vi "模块启用配置框.vi"() -> ()   [LabVIEW 2022 SP3]
uses:
  <vilib>/Utility/config.llb/NI_LVConfig.lvlib
  <userlib>/_OpenG.lib/variantconfig/variantconfig.llb/openg_variant_configuration_file.lvlib
panel:
  in  "旁路系统启用":bool caption="启用"
  in  "综合生物毒性启用":bool caption="启用"
  in  "雷达流速仪启用":bool caption="启用"
  in  "ADCP启用":bool caption="启用"
  in  "挥发酚启用":bool caption="启用"
  in  "重金属启用":bool caption="启用"
  in  "运维打卡启用":bool caption="启用"
  in  "氟化物连接配置":T1={"启用"=FALSE, "连接类型"=enum."串口", "串口"="", "波特率"=115200, "IP"="", "PORT"="502"} {"波特率" items=["115200"=115200, "9600"=9600]}
  in  "加标回收模块版本":T2=enum."V4"
  in  "多参数模块版本":T3=enum."集成式多参"
  in  "总氮模块版本":T4=enum."V3"
  in  "总磷模块版本":T4=enum."V3"
  in  "加标回收连接配置":T1={"启用"=FALSE, "连接类型"=enum."串口", "串口"="", "波特率"=115200, "IP"="", "PORT"="502"} {"波特率" items=["115200"=115200, "9600"=9600]}
  in  "多参数连接配置":T1={"启用"=FALSE, "连接类型"=enum."串口", "串口"="", "波特率"=115200, "IP"="", "PORT"="502"} {"波特率" items=["115200"=115200, "9600"=9600]}
  in  "CODcr连接配置":T1={"启用"=FALSE, "连接类型"=enum."串口", "串口"="", "波特率"=115200, "IP"="", "PORT"="502"} {"波特率" items=["115200"=115200, "9600"=9600]}
  in  "CODMn连接配置":T1={"启用"=FALSE, "连接类型"=enum."串口", "串口"="", "波特率"=115200, "IP"="", "PORT"="502"} {"波特率" items=["115200"=115200, "9600"=9600]}
  in  "总氮连接配置":T1={"启用"=FALSE, "连接类型"=enum."串口", "串口"="", "波特率"=115200, "IP"="", "PORT"="502"} {"波特率" items=["115200"=115200, "9600"=9600]}
  in  "总磷连接配置":T1={"启用"=FALSE, "连接类型"=enum."串口", "串口"="", "波特率"=115200, "IP"="", "PORT"="502"} {"波特率" items=["115200"=115200, "9600"=9600]}
  in  "氨氮连接配置":T1={"启用"=FALSE, "连接类型"=enum."串口", "串口"="", "波特率"=115200, "IP"="", "PORT"="502"} {"波特率" items=["115200"=115200, "9600"=9600]}
  in  "进样类型":T5={"氨氮采样杯采样"=TRUE, "总磷采样杯采样"=TRUE, "总氮采样杯采样"=TRUE, "CODMn采样杯采样"=TRUE, "CODcr采样杯采样"=TRUE, "氟化物采样杯采样"=TRUE, "挥发酚采样杯采样"=TRUE}
  in  "CODcr模块版本":T6
  in  "加载配置":bool
  in  "河水净化启用":bool caption="启用"
  in  "流量计启用":bool caption="启用"
  in  "超标留样启用":bool caption="启用"
  in  "氨氮模块版本":T4=enum."V3"
  in  "设备类型":T7=enum."浮船"
  in  "采配水模块类型":T8=enum."V4"
  in  "CODMn模块版本":T9
  in  "数据库类型":T10
  in  "模块配置类型":T11
  in  "取消":bool
  in  "确认":bool
  # "模块启用配置"
  # "说明:\n选择所需要启动的模块,并按确认,软件将重启生效."
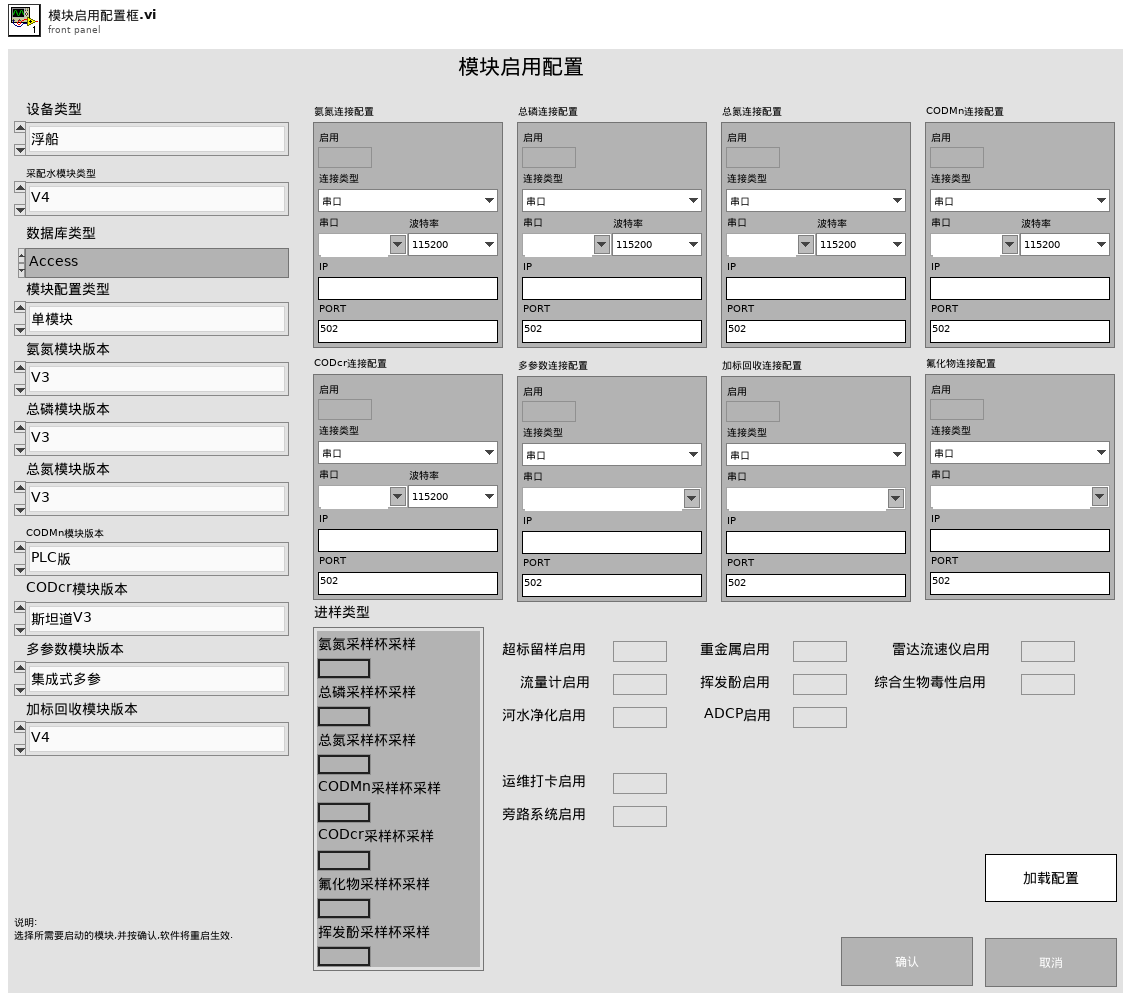
[diagram p1: front panel]
types:
  T1 = typedef "连接配置.ctl" = cluster{"启用":bool, "连接类型":enum16{"串口", "TCP"}, "串口":string, "波特率":u32, "IP":string, "PORT":string}
  T2 = typedef "加标回收模块版本.ctl" = enum16{"V1", "V2", "V4"}
  T3 = typedef "多参数模块版本.ctl" = enum16{"原位多参数", "集成式多参"}
  T4 = typedef "氨氮总磷总氮模块版本.ctl" = enum16{"V2", "V3"}
  T5 = cluster{"氨氮采样杯采样":bool, "总磷采样杯采样":bool, "总氮采样杯采样":bool, "CODMn采样杯采样":bool, "CODcr采样杯采样":bool, "氟化物采样杯采样":bool, "挥发酚采样杯采样":bool}
  T6 = typedef "CODcr模块版本.ctl" = enum16{"斯坦道V3", "点创"}
  T7 = typedef "设备类型.ctl" = enum16{"微站", "固定站", "浮船"}
  T8 = typedef "采配水类型.ctl" = enum16{"V1", "V2", "V3", "V4", "室内V1", "室内V2", "固定站V1", "固定站V2", "浮船V1", "浮船V2", "养殖尾水", "广东华南所"}
  T9 = typedef "CODMn模块版本.ctl" = enum16{"PLC版", "单片机版", "通用流路版本"}
  T10 = typedef "数据库类型.ctl" = enum16{"Access", "SQLite"}
  T11 = typedef "模块配置类型.ctl" = enum16{"单模块", "总磷总氮二合一模块", "氨氮总磷二合一模块"}
  T12 = cluster{"氨氮采样杯采样":bool, "总磷采样杯采样":bool, "总氮采样杯采样":bool, "CODMn采样杯采样":bool, "CODcr采样杯采样":bool, "氟化物采样杯采样":bool, "氟化物采样杯采样 2":bool}
  T13 = cluster{"总磷总氮启用":bool, "MB通信方式选择":enum16{"串口", "TCP"}, "VISA Resource":refnum<visa-resource-name>, "波特率":u32, "IP":string, "PORT":string}
  T14 = cluster{"质控单元启用":bool, u16, "COM Port":refnum<visa-resource-name>, "Baud Rate (bps)":u32, "IP Address":string, string}
  T15 = cluster{"氟化物启用":bool, "MB通信方式选择":enum16{"串口", "TCP"}, "VISA Resource":refnum<visa-resource-name>, "波特率":u32, "IP":string, "PORT":string}
  T16 = cluster{"总氮启用":bool, "MB通信方式选择":enum16{"串口", "TCP"}, "VISA Resource":refnum<visa-resource-name>, "波特率":u32, "IP":string, "PORT":string}
  T17 = cluster{"多参数启用":bool, "MB通信方式选择":enum16{"串口", "TCP"}, "VISA Resource":refnum<visa-resource-name>, "波特率":u32, "IP":string, "PORT":string}
  T18 = cluster{"多参数启用":bool, "连接方式":u16, "VISA资源名称":refnum<visa-resource-name>, "波特率":u32, "IP":string, string}
  T19 = cluster{"氨氮启用":bool, "MB通信方式选择":enum16{"串口", "TCP"}, "VISA Resource":refnum<visa-resource-name>, "波特率":u32, "IP":string, "PORT":string}
  T20 = cluster{"CODcr启用":bool, "MB通信方式选择":enum16{"串口", "TCP"}, "VISA Resource":refnum<visa-resource-name>, "波特率":u32, "IP":string, "PORT":string}
  T21 = cluster{"baud rate (bps)":u32, "stop bits":u16, "parity":u16, "flow control":u16, "timeout":u32, "retries":i32}
  T22 = cluster{"CODMn启用":bool, "MB通信方式选择":enum16{"串口", "TCP"}, "VISA resource name":refnum<visa-resource-name>, "baud rate (bps)":u32, "IP":string, "PORT":string}
  T23 = cluster{"CODMn启用":bool, "MB通信方式选择":enum16{"串口", "TCP"}, "VISA Resource":refnum<visa-resource-name>, "波特率":u32, "IP":string, "PORT":string}
  T24 = typedef "配置表选择.ctl" = enum16{"微站常规九参总磷总氮二合一", "微站常规八参氨氮总磷二合一", "微站常规九参", "微站常规八参", "固定站常规九参（TCP连接）", "固定站常规九参（串口连接）", "浮船常规九参总磷总氮二合一", "浮船常规九参"}
  T25 = typedef "模块配置表.ctl" = cluster{"设备类型":T7, "采配水模块类型":T8, "数据库类型":T10, "模块配置类型":T11, "氨氮模块版本":T4, "总磷模块版本":T4, "总氮模块版本":T4, "CODMn模块版本":T9, "CODcr模块版本":T6, "多参数模块版本":T3, "加标回收模块版本":T2, "氨氮连接配置":T1, "总磷连接配置":T1, "总氮连接配置":T1, "CODMn连接配置":T1, "CODcr连接配置":T1, "多参数连接配置":T1, "加标回收连接配置":T1, "超标留样启用":bool, "流量计启用":bool, "河水净化启用":bool, "进样类型":cluster{"氨氮采样杯采样":bool, "总磷采样杯采样":bool, "总氮采样杯采样":bool, "CODMn采样杯采样":bool, "CODcr采样杯采样":bool, "氟化物采样杯采样":bool, "挥发酚采样杯采样":bool}, "氟化物连接配置":T1}
  T26 = typedef "NI_LVConfig.lvlib/Config Data RefNum.ctl" = refnum<k1>
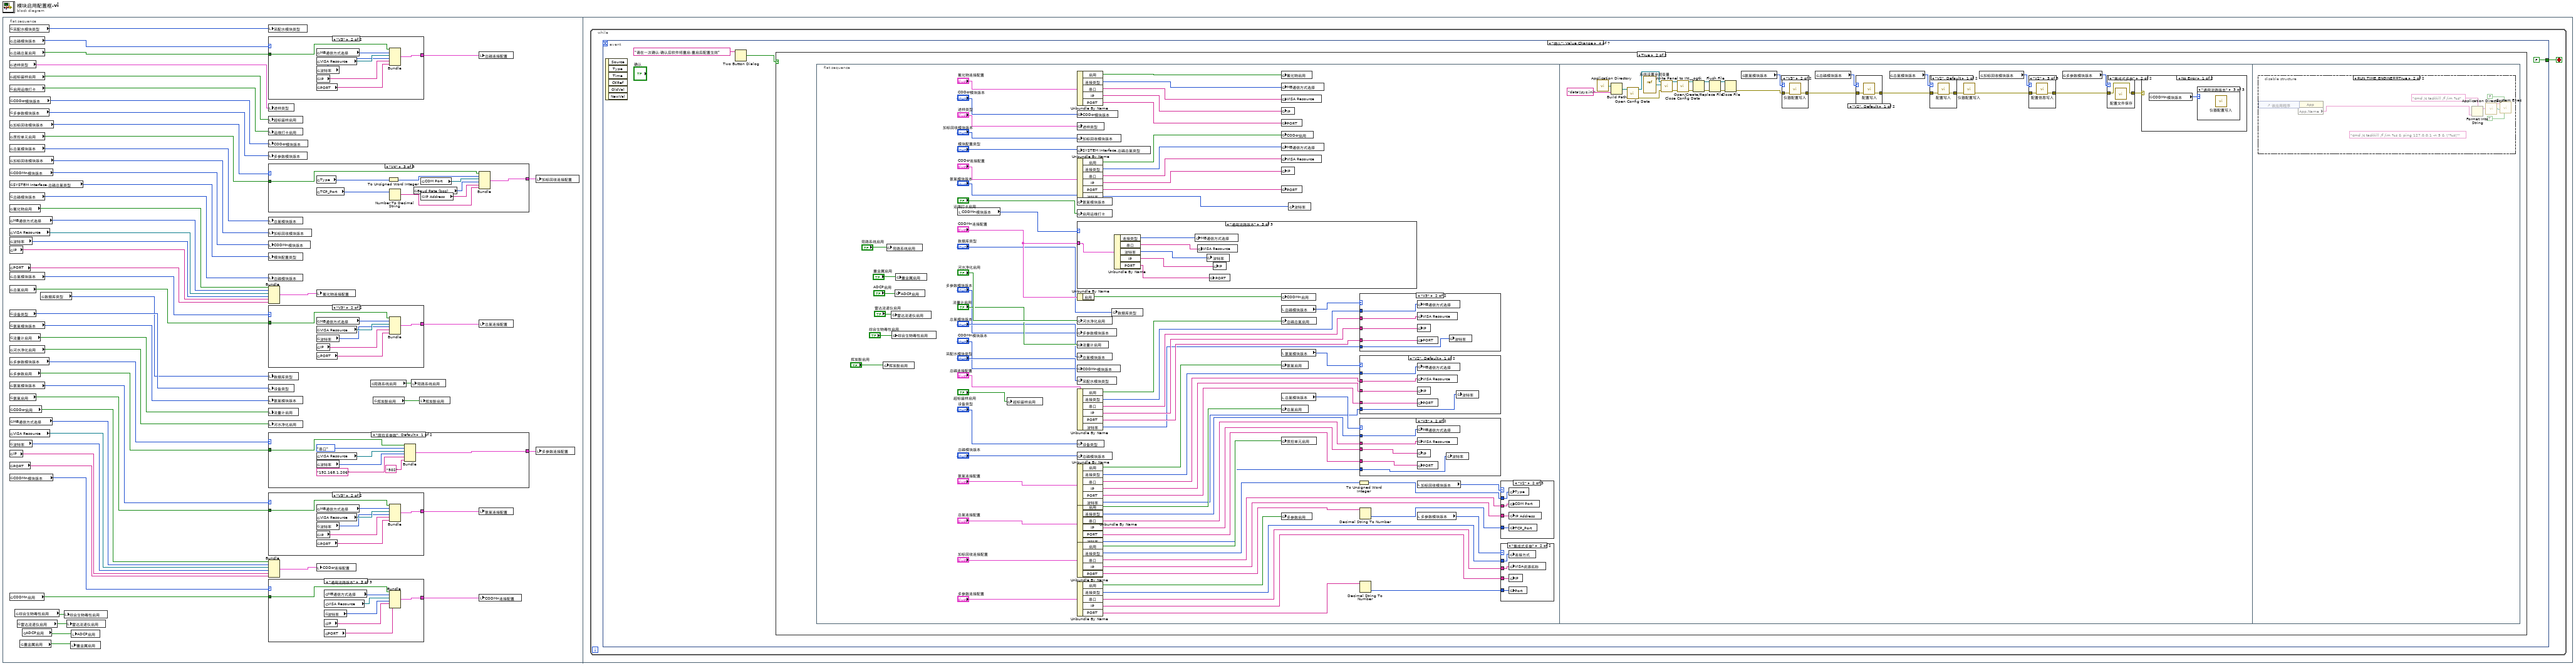
[diagram p0: block diagram]
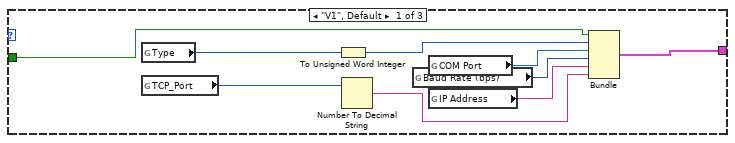
[diagram p2: hidden frame]
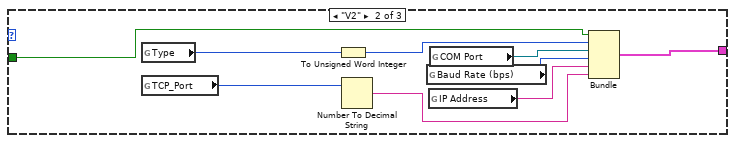
[diagram p3: hidden frame]
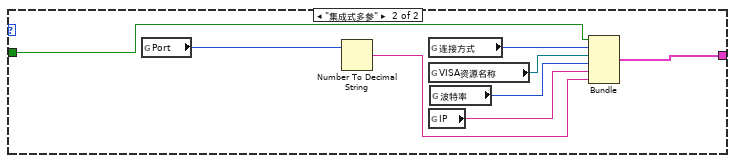
[diagram p4: hidden frame]
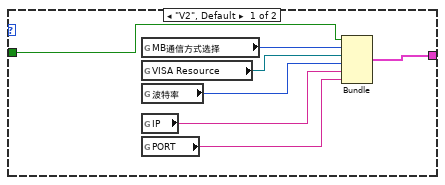
[diagram p5: hidden frame]
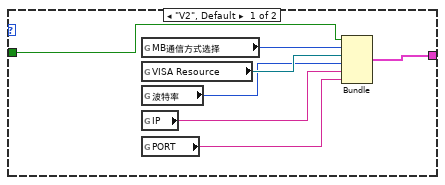
[diagram p6: hidden frame]
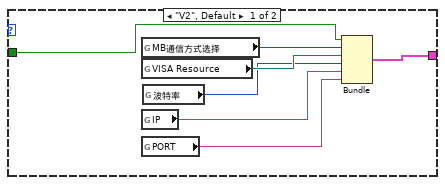
[diagram p7: hidden frame]
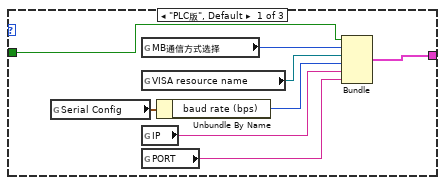
[diagram p8: hidden frame]
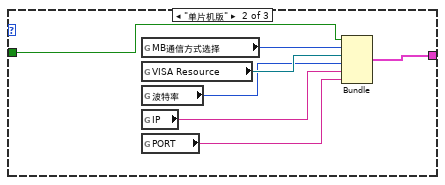
[diagram p9: hidden frame]
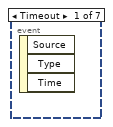
[diagram p10: hidden frame]
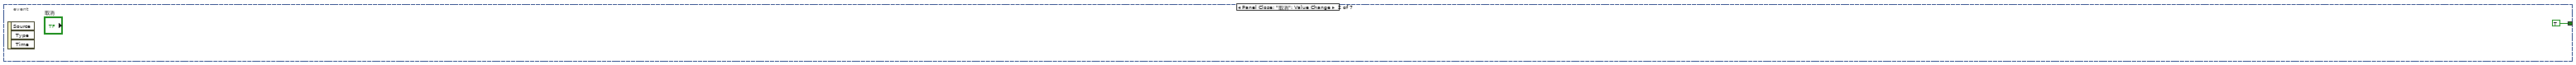
[diagram p11: hidden frame]
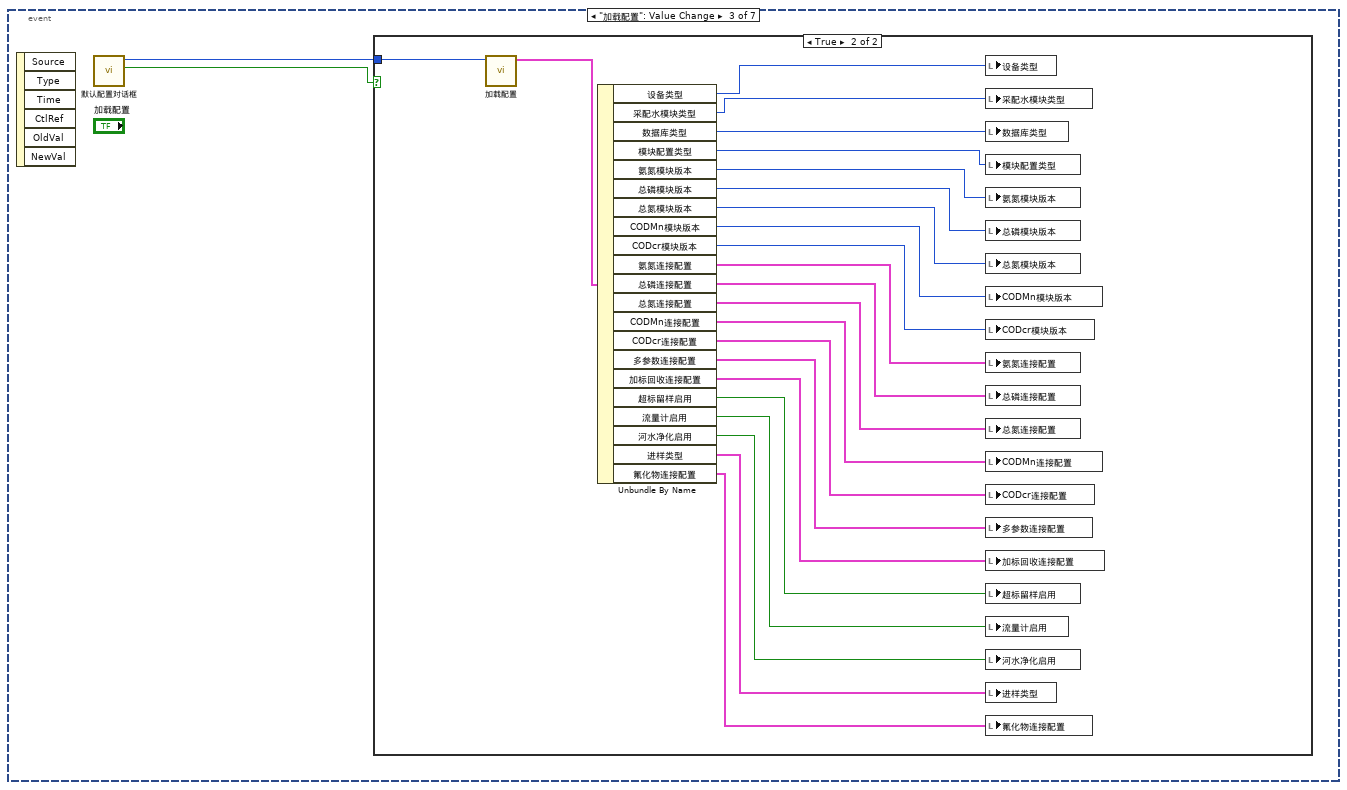
[diagram p12: hidden frame]
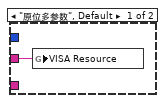
[diagram p15: hidden frame]
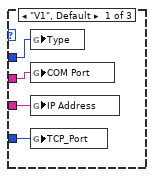
[diagram p16: hidden frame]
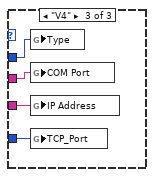
[diagram p17: hidden frame]
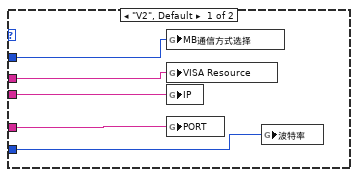
[diagram p18: hidden frame]
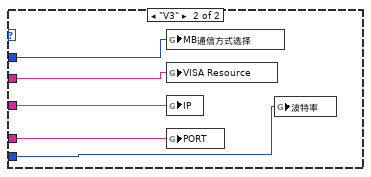
[diagram p19: hidden frame]
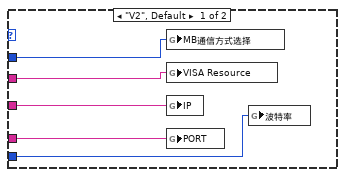
[diagram p20: hidden frame]
diagram:
  n1 = flat-sequence {
    frame #0 {
      n2 = global read "系统设置全局变量.vi" "采配水模块类型"() -> (w53:T8)
      n3 = global read "系统设置全局变量.vi" "总磷模块版本"() -> (w27:T4)
      n4 = global read "系统设置全局变量.vi" "总磷总氮启用"() -> (w25:bool)
      n5 = global read "系统设置全局变量.vi" "进样类型"() -> (w48:T5)
      n6 = global read "系统设置全局变量.vi" "超标留样启用"() -> (w47:bool)
      n7 = global read "系统设置全局变量.vi" "启用运维打卡"() -> (w11:bool)
      n8 = global read "系统设置全局变量.vi" "CODcr模块版本"() -> (w49:T6)
      n9 = global read "系统设置全局变量.vi" "多参数模块版本"() -> (w23:T3)
      n10 = global read "系统设置全局变量.vi" "加标回收模块版本"() -> (w19:T2)
      n11 = global read "系统设置全局变量.vi" "质控单元启用"() -> (w18:bool)
      n12 = global read "系统设置全局变量.vi" "总氮模块版本"() -> (w30:T4)
      n13 = global read "系统设置全局变量.vi" "加标回收模块版本"() -> (w20:T2)
      n14 = global read "系统设置全局变量.vi" "CODMn模块版本"() -> (w50:T9)
      n15 = global read "系统设置全局变量.vi" "SYSTEM Interface.总磷总氮类型"() -> (w52:T11)
      n16 = global read "系统设置全局变量.vi" "总磷模块版本"() -> (w31:T4)
      n17 = global read "系统设置全局变量.vi" "氟化物启用"() -> (w13:bool)
      n18 = global read "总磷总氮断电保存全局变量.vi" "MB通信方式选择"() -> (w14:enum16{"串口", "TCP"})
      n19 = global read "总磷总氮断电保存全局变量.vi" "VISA Resource"() -> (w15:refnum<visa-resource-name>)
      n20 = global read "总磷总氮断电保存全局变量.vi" "波特率"() -> (w4:u32)
      n21 = global read "总磷总氮断电保存全局变量.vi" "IP"() -> (w16:string)
      n22 = global read "总磷总氮断电保存全局变量.vi" "PORT"() -> (w17:string)
      n23 = global read "系统设置全局变量.vi" "总氮模块版本"() -> (w26:T4)
      n24 = global read "系统设置全局变量.vi" "总氮启用"() -> (w24:bool)
      n25 = global read "系统设置全局变量.vi" "设备类型"() -> (w54:T7)
      n26 = global read "系统设置全局变量.vi" "氨氮模块版本"() -> (w51:T4)
      n27 = global read "系统设置全局变量.vi" "流量计启用"() -> (w46:bool)
      n28 = global read "系统设置全局变量.vi" "河水净化启用"() -> (w45:bool)
      n29 = global read "系统设置全局变量.vi" "多参数模块版本"() -> (w22:T3)
      n30 = global read "系统设置全局变量.vi" "多参数启用"() -> (w21:bool)
      n31 = global read "系统设置全局变量.vi" "氨氮模块版本"() -> (w29:T4)
      n32 = global read "系统设置全局变量.vi" "氨氮启用"() -> (w28:bool)
      n33 = global read "系统设置全局变量.vi" "CODcr启用"() -> (w38:bool)
      n34 = global read "总磷总氮断电保存全局变量.vi" "MB通信方式选择"() -> (w37:enum16{"串口", "TCP"})
      n35 = global read "总磷总氮断电保存全局变量.vi" "VISA Resource"() -> (w6:refnum<visa-resource-name>)
      n36 = global read "总磷总氮断电保存全局变量.vi" "波特率"() -> (w5:u32)
      n37 = global read "总磷总氮断电保存全局变量.vi" "IP"() -> (w36:string)
      n38 = global read "总磷总氮断电保存全局变量.vi" "PORT"() -> (w35:string)
      n39 = global read "系统设置全局变量.vi" "CODMn模块版本"() -> (w41:T9)
      n40 = global read "系统设置全局变量.vi" "CODMn启用"() -> (w40:bool)
      n41 = global read "系统设置全局变量.vi" "综合生物毒性启用"() -> (w3:bool)
      n42 = global read "系统设置全局变量.vi" "雷达流速仪启用"() -> (w1:bool)
      n43 = global read "系统设置全局变量.vi" "重金属启用"() -> (w10:bool)
      n44 = global read "系统设置全局变量.vi" "ADCP启用"() -> (w7:bool)
      n45 = global read "非断电保持全局变量.vi" "数据库类型"() -> (w8:T10)
      n46 = local write "综合生物毒性启用"(w3) -> ()
      n47 = local write "雷达流速仪启用"(w1) -> ()
      n48 = local write "重金属启用"(w10) -> ()
      n49 = local write "ADCP启用"(w7) -> ()
      n50 = local write "采配水模块类型"(w53) -> ()
      n51 = case shown="\"V3\"" w27 {
        tunnel: [w112 w120] -> w43
        tunnel: w25 -> [w117 w119]
        frame "V2", Default {
          n52 = global read "总磷总氮断电保存全局变量.vi" "MB通信方式选择"() -> (w116:enum16{"串口", "TCP"})
          n53 = global read "总磷总氮断电保存全局变量.vi" "VISA Resource"() -> (w115:refnum<visa-resource-name>)
          n54 = global read "总磷总氮断电保存全局变量.vi" "波特率"() -> (w111:u32)
          n55 = global read "总磷总氮断电保存全局变量.vi" "IP"() -> (w114:string)
          n56 = global read "总磷总氮断电保存全局变量.vi" "PORT"() -> (w113:string)
          n57 = Bundle("总磷总氮启用"=w117, "MB通信方式选择"=w116, "VISA Resource"=w115, "波特率"=w111, "IP"=w114, "PORT"=w113) -> (w112:T13)  [unwired: 1 in]
        }
        frame "V3" {
          n58 = global read "总磷总氮断电保存全局变量.vi" "MB通信方式选择"() -> (w124:enum16{"串口", "TCP"})
          n59 = global read "总磷总氮断电保存全局变量.vi" "VISA Resource"() -> (w123:refnum<visa-resource-name>)
          n60 = global read "总磷总氮断电保存全局变量.vi" "波特率"() -> (w118:u32)
          n61 = global read "总磷总氮断电保存全局变量.vi" "IP"() -> (w122:string)
          n62 = global read "总磷总氮断电保存全局变量.vi" "PORT"() -> (w121:string)
          n63 = Bundle("总磷总氮启用"=w119, "MB通信方式选择"=w124, "VISA Resource"=w123, "波特率"=w118, "IP"=w122, "PORT"=w121) -> (w120:T13)  [unwired: 1 in]
        }
      }
      n64 = local write "进样类型"(w48) -> ()
      n65 = local write "超标留样启用"(w47) -> ()
      n66 = local write "运维打卡启用"(w11) -> ()
      n67 = local write "CODcr模块版本"(w49) -> ()
      n68 = local write "多参数模块版本"(w23) -> ()
      n69 = case shown="\"V4\"" w19 {
        tunnel: [w62 w71 w77] -> w32
        tunnel: w18 -> [w63 w72 w74]
        frame "V1", Default {
          n70 = global read "ZK断电保存全局变量.vi" "Type"() -> (w61:enum16{"Serial", "TCP"})
          n71 = global read "ZK断电保存全局变量.vi" "TCP_Port"() -> (w57:u16)
          n72 = To Unsigned Word Integer(number=w61) -> (unsigned 16bit integer=w60:u16)
          n73 = Number To Decimal String(number=w57) -> (decimal integer string=w56:string)  [unwired: 1 in]
          n74 = global read "ZK断电保存全局变量.vi" "Baud Rate (bps)"() -> (w55:u32)
          n75 = global read "ZK断电保存全局变量.vi" "COM Port"() -> (w59:refnum<visa-resource-name>)
          n76 = global read "ZK断电保存全局变量.vi" "IP Address"() -> (w58:string)
          n77 = Bundle("质控单元启用"=w63, w60, "COM Port"=w59, "Baud Rate (bps)"=w55, "IP Address"=w58, w56) -> (w62:T14)  [unwired: 1 in]
        }
        frame "V2" {
          n78 = global read "ZK断电保存全局变量.vi" "Type"() -> (w68:enum16{"Serial", "TCP"})
          n79 = global read "ZK断电保存全局变量.vi" "TCP_Port"() -> (w65:u16)
          n80 = To Unsigned Word Integer(number=w68) -> (unsigned 16bit integer=w70:u16)
          n81 = Number To Decimal String(number=w65) -> (decimal integer string=w69:string)  [unwired: 1 in]
          n82 = global read "ZK断电保存全局变量.vi" "Baud Rate (bps)"() -> (w64:u32)
          n83 = global read "ZK断电保存全局变量.vi" "IP Address"() -> (w66:string)
          n84 = global read "ZK断电保存全局变量.vi" "COM Port"() -> (w67:refnum<visa-resource-name>)
          n85 = Bundle("质控单元启用"=w72, w70, "COM Port"=w67, "Baud Rate (bps)"=w64, "IP Address"=w66, w69) -> (w71:T14)  [unwired: 1 in]
        }
        frame "V4" {
          n86 = global read "ZK断电保存全局变量.vi" "Type"() -> (w80:enum16{"Serial", "TCP"})
          n87 = global read "ZK断电保存全局变量.vi" "TCP_Port"() -> (w81:u16)
          n88 = To Unsigned Word Integer(number=w80) -> (unsigned 16bit integer=w75:u16)
          n89 = Number To Decimal String(number=w81) -> (decimal integer string=w76:string)  [unwired: 1 in]
          n90 = global read "ZK断电保存全局变量.vi" "Baud Rate (bps)"() -> (w73:u32)
          n91 = global read "ZK断电保存全局变量.vi" "COM Port"() -> (w79:refnum<visa-resource-name>)
          n92 = global read "ZK断电保存全局变量.vi" "IP Address"() -> (w78:string)
          n93 = Bundle("质控单元启用"=w74, w75, "COM Port"=w79, "Baud Rate (bps)"=w73, "IP Address"=w78, w76) -> (w77:T14)  [unwired: 1 in]
        }
      }
      n94 = local write "总氮模块版本"(w30) -> ()
      n95 = local write "加标回收模块版本"(w20) -> ()
      n96 = local write "CODMn模块版本"(w50) -> ()
      n97 = local write "模块配置类型"(w52) -> ()
      n98 = local write "总磷模块版本"(w31) -> ()
      n99 = Bundle("氟化物启用"=w13, "MB通信方式选择"=w14, "VISA Resource"=w15, "波特率"=w4, "IP"=w16, "PORT"=w17) -> (w12:T15)  [unwired: 1 in]
      n100 = case shown="\"V3\"" w26 {
        tunnel: [w101 w106] -> w42
        tunnel: w24 -> [w103 w105]
        frame "V2", Default {
          n101 = global read "总磷总氮断电保存全局变量.vi" "MB通信方式选择"() -> (w102:enum16{"串口", "TCP"})
          n102 = global read "总磷总氮断电保存全局变量.vi" "VISA Resource"() -> (w100:refnum<visa-resource-name>)
          n103 = global read "总磷总氮断电保存全局变量.vi" "波特率"() -> (w97:u32)
          n104 = global read "总磷总氮断电保存全局变量.vi" "IP"() -> (w99:string)
          n105 = global read "总磷总氮断电保存全局变量.vi" "PORT"() -> (w98:string)
          n106 = Bundle("总氮启用"=w103, "MB通信方式选择"=w102, "VISA Resource"=w100, "波特率"=w97, "IP"=w99, "PORT"=w98) -> (w101:T16)  [unwired: 1 in]
        }
        frame "V3" {
          n107 = global read "总磷总氮断电保存全局变量.vi" "MB通信方式选择"() -> (w110:enum16{"串口", "TCP"})
          n108 = global read "总磷总氮断电保存全局变量.vi" "VISA Resource"() -> (w109:refnum<visa-resource-name>)
          n109 = global read "总磷总氮断电保存全局变量.vi" "波特率"() -> (w104:u32)
          n110 = global read "总磷总氮断电保存全局变量.vi" "IP"() -> (w108:string)
          n111 = global read "总磷总氮断电保存全局变量.vi" "PORT"() -> (w107:string)
          n112 = Bundle("总氮启用"=w105, "MB通信方式选择"=w110, "VISA Resource"=w109, "波特率"=w104, "IP"=w108, "PORT"=w107) -> (w106:T16)  [unwired: 1 in]
        }
      }
      n113 = local write "数据库类型"(w8) -> ()
      n114 = local write "设备类型"(w54) -> ()
      n115 = local write "氨氮模块版本"(w51) -> ()
      n116 = local write "流量计启用"(w46) -> ()
      n117 = local write "河水净化启用"(w45) -> ()
      n118 = case shown="\"原位多参数\", Default" w22 {
        tunnel: [w83 w93] -> w33
        tunnel: w21 -> [w88 w90]
        frame "原位多参数", Default {
          n119 = global read "多参数断电保存全局变量.vi" "VISA Resource"() -> (w87:refnum<visa-resource-name>)
          n120 = global read "多参数断电保存全局变量.vi" "波特率"() -> (w82:u32)
          n121 = Bundle("多参数启用"=w88, "MB通信方式选择"=enum16{"串口", "TCP"}."串口", "VISA Resource"=w87, "波特率"=w82, "IP"="192.168.1.206", "PORT"="502") -> (w83:T17)  [unwired: 1 in]
        }
        frame "集成式多参" {
          n122 = global read "断电保存变量.vi" "Port"() -> (w92:u16)
          n123 = Number To Decimal String(number=w92) -> (decimal integer string=w91:string)  [unwired: 1 in]
          n124 = global read "断电保存变量.vi" "连接方式"() -> (w96:u16)
          n125 = global read "断电保存变量.vi" "VISA资源名称"() -> (w95:refnum<visa-resource-name>)
          n126 = global read "断电保存变量.vi" "IP"() -> (w94:string)
          n127 = global read "断电保存变量.vi" "波特率"() -> (w89:u32)
          n128 = Bundle("多参数启用"=w90, "连接方式"=w96, "VISA资源名称"=w95, "波特率"=w89, "IP"=w94, w91) -> (w93:T18)  [unwired: 1 in]
        }
      }
      n129 = case shown="\"V3\"" w29 {
        tunnel: [w130 w134] -> w44
        tunnel: w28 -> [w131 w133]
        frame "V2", Default {
          n130 = global read "总磷总氮断电保存全局变量.vi" "MB通信方式选择"() -> (w129:enum16{"串口", "TCP"})
          n131 = global read "总磷总氮断电保存全局变量.vi" "VISA Resource"() -> (w128:refnum<visa-resource-name>)
          n132 = global read "总磷总氮断电保存全局变量.vi" "IP"() -> (w127:string)
          n133 = global read "总磷总氮断电保存全局变量.vi" "PORT"() -> (w126:string)
          n134 = global read "总磷总氮断电保存全局变量.vi" "波特率"() -> (w125:u32)
          n135 = Bundle("氨氮启用"=w131, "MB通信方式选择"=w129, "VISA Resource"=w128, "波特率"=w125, "IP"=w127, "PORT"=w126) -> (w130:T19)  [unwired: 1 in]
        }
        frame "V3" {
          n136 = global read "总磷总氮断电保存全局变量.vi" "MB通信方式选择"() -> (w138:enum16{"串口", "TCP"})
          n137 = global read "总磷总氮断电保存全局变量.vi" "VISA Resource"() -> (w137:refnum<visa-resource-name>)
          n138 = global read "总磷总氮断电保存全局变量.vi" "波特率"() -> (w132:u32)
          n139 = global read "总磷总氮断电保存全局变量.vi" "IP"() -> (w136:string)
          n140 = global read "总磷总氮断电保存全局变量.vi" "PORT"() -> (w135:string)
          n141 = Bundle("氨氮启用"=w133, "MB通信方式选择"=w138, "VISA Resource"=w137, "波特率"=w132, "IP"=w136, "PORT"=w135) -> (w134:T19)  [unwired: 1 in]
        }
      }
      n142 = Bundle("CODcr启用"=w38, "MB通信方式选择"=w37, "VISA Resource"=w6, "波特率"=w5, "IP"=w36, "PORT"=w35) -> (w34:T20)  [unwired: 1 in]
      n143 = case shown="\"通用流路版本\"" w41 {
        tunnel: w40 -> [w146 w152 w160]
        tunnel: [w144 w148 w159] -> w39
        frame "PLC版", Default {
          n144 = global read "CODMn断电保存全局变量.vi" "Serial Config"() -> (w140:T21)
          n145 = global read "CODMn断电保存全局变量.vi" "MB通信方式选择"() -> (w145:enum16{"串口", "TCP"})
          n146 = global read "CODMn断电保存全局变量.vi" "VISA resource name"() -> (w143:refnum<visa-resource-name>)
          n147 = global read "CODMn断电保存全局变量.vi" "IP"() -> (w142:string)
          n148 = global read "CODMn断电保存全局变量.vi" "PORT"() -> (w141:string)
          n149 = Unbundle By Name(w140) -> ("baud rate (bps)"=w139:u32)
          n150 = Bundle("CODMn启用"=w146, "MB通信方式选择"=w145, "VISA resource name"=w143, "baud rate (bps)"=w139, "IP"=w142, "PORT"=w141) -> (w144:T22)  [unwired: 1 in]
        }
        frame "单片机版" {
          n151 = global read "CODMn断电保存全局变量.vi" "MB通信方式选择"() -> (w153:enum16{"串口", "TCP"})
          n152 = global read "CODMn断电保存全局变量.vi" "VISA Resource"() -> (w151:refnum<visa-resource-name>)
          n153 = global read "CODMn断电保存全局变量.vi" "波特率"() -> (w147:u32)
          n154 = global read "CODMn断电保存全局变量.vi" "IP"() -> (w150:string)
          n155 = global read "CODMn断电保存全局变量.vi" "PORT"() -> (w149:string)
          n156 = Bundle("CODMn启用"=w152, "MB通信方式选择"=w153, "VISA Resource"=w151, "波特率"=w147, "IP"=w150, "PORT"=w149) -> (w148:T23)  [unwired: 1 in]
        }
        frame "通用流路版本" {
          n157 = global read "总磷总氮断电保存全局变量.vi" "MB通信方式选择"() -> (w158:enum16{"串口", "TCP"})
          n158 = global read "总磷总氮断电保存全局变量.vi" "VISA Resource"() -> (w157:refnum<visa-resource-name>)
          n159 = global read "总磷总氮断电保存全局变量.vi" "波特率"() -> (w156:u32)
          n160 = global read "总磷总氮断电保存全局变量.vi" "IP"() -> (w155:string)
          n161 = global read "总磷总氮断电保存全局变量.vi" "PORT"() -> (w154:string)
          n162 = Bundle("CODMn启用"=w160, "MB通信方式选择"=w158, "VISA Resource"=w157, "波特率"=w156, "IP"=w155, "PORT"=w154) -> (w159:T23)  [unwired: 1 in]
        }
      }
      n163 = local write "氟化物连接配置"(w12) -> ()
      n164 = local write "CODcr连接配置"(w34) -> ()
      n165 = global read "系统设置全局变量.vi" "旁路系统启用"() -> (w2:bool)
      n166 = global read "系统设置全局变量.vi" "挥发酚启用"() -> (w9:bool)
      n167 = local write "旁路系统启用"(w2) -> ()
      n168 = local write "挥发酚启用"(w9) -> ()
      n169 = local write "总磷连接配置"(w43) -> ()
      n170 = local write "总氮连接配置"(w42) -> ()
      n171 = local write "氨氮连接配置"(w44) -> ()
      n172 = local write "CODMn连接配置"(w39) -> ()
      n173 = local write "加标回收连接配置"(w32) -> ()
      n174 = local write "多参数连接配置"(w33) -> ()
    }
    frame #1 {
      n175 = while {
        stop <- w161 stop-if-true
        n176 = event shown="[3] \"确认\": Value Change" {
          selector: _ -> [_ _ _ _ _ _ _]
          dyn-events: _ -> [_ _ _ _ _ _ _]
          timeout: _ -> [_ _ _ _ _ _ _]
          tunnel: [_ TRUE _ FALSE _ _ _] -> w161
          event Timeout {
            n177 = event-data() -> ()  [unwired: 1 in, 3 out]
          }
          event Panel Close; "取消": Value Change {
            n178 = event-data() -> ()  [unwired: 1 in, 3 out]
          }
          event "加载配置": Value Change {
            n179 = event-data() -> ()  [unwired: 1 in, 6 out]
            n180 = call "默认配置对话框.vi"() -> ("check？"=w163:bool, "默认配置选择输出"=w164:T24)  [unwired: 10 in]
            n181 = case shown="True" w163 {
              tunnel: w164 -> [_ w187]
              frame False {
              }
              frame True {
                n182 = call "加载配置.vi"("默认配置选择"=w187) -> ("配置表"=w186:T25)  [unwired: 10 in]
                n183 = Unbundle By Name(w186) -> ("设备类型"=w185:T7, "采配水模块类型"=w184:T8, "数据库类型"=w183:T10, "模块配置类型"=w182:T11, "氨氮模块版本"=w181:T4, "总磷模块版本"=w166:T4, "总氮模块版本"=w167:T4, "CODMn模块版本"=w180:T9, "CODcr模块版本"=w179:T6, "氨氮连接配置"=w178:T1, "总磷连接配置"=w177:T1, "总氮连接配置"=w176:T1, "CODMn连接配置"=w175:T1, "CODcr连接配置"=w174:T1, "多参数连接配置"=w173:T1, "加标回收连接配置"=w172:T1, "超标留样启用"=w171:bool, "流量计启用"=w170:bool, "河水净化启用"=w169:bool, "进样类型"=w168:T5, "氟化物连接配置"=w165:T1)
                n184 = local write "设备类型"(w185) -> ()
                n185 = local write "采配水模块类型"(w184) -> ()
                n186 = local write "数据库类型"(w183) -> ()
                n187 = local write "模块配置类型"(w182) -> ()
                n188 = local write "氨氮模块版本"(w181) -> ()
                n189 = local write "总磷模块版本"(w166) -> ()
                n190 = local write "总氮模块版本"(w167) -> ()
                n191 = local write "CODMn模块版本"(w180) -> ()
                n192 = local write "CODcr模块版本"(w179) -> ()
                n193 = local write "氨氮连接配置"(w178) -> ()
                n194 = local write "总磷连接配置"(w177) -> ()
                n195 = local write "总氮连接配置"(w176) -> ()
                n196 = local write "CODMn连接配置"(w175) -> ()
                n197 = local write "CODcr连接配置"(w174) -> ()
                n198 = local write "多参数连接配置"(w173) -> ()
                n199 = local write "加标回收连接配置"(w172) -> ()
                n200 = local write "超标留样启用"(w171) -> ()
                n201 = local write "流量计启用"(w170) -> ()
                n202 = local write "河水净化启用"(w169) -> ()
                n203 = local write "进样类型"(w168) -> ()
                n204 = local write "氟化物连接配置"(w165) -> ()
              }
            }
          }
          event "确认": Value Change {
            n205 = event-data() -> ()  [unwired: 1 in, 6 out]
            n206 = Two Button Dialog(message="请在一次确认,确认后软件将重启,重启后配置生效" ("消息")) -> (T button?=w188:bool)  [unwired: 2 in]
            n207 = case shown="True" w188 {
              frame False {
              }
              frame True {
                n208 = flat-sequence {
                  frame #0 {
                    n209 = global write "系统设置全局变量.vi" "挥发酚启用"("挥发酚启用") -> ()
                    n210 = global write "系统设置全局变量.vi" "旁路系统启用"("旁路系统启用") -> ()
                    n211 = global write "系统设置全局变量.vi" "雷达流速仪启用"("雷达流速仪启用") -> ()
                    n212 = global write "系统设置全局变量.vi" "综合生物毒性启用"("综合生物毒性启用") -> ()
                    n213 = global write "系统设置全局变量.vi" "ADCP启用"("ADCP启用") -> ()
                    n214 = global write "系统设置全局变量.vi" "重金属启用"("重金属启用") -> ()
                    n215 = local read "CODMn模块版本"() -> (w247:T9)
                    n216 = global write "系统设置全局变量.vi" "超标留样启用"("超标留样启用") -> ()
                    n217 = Unbundle By Name("氟化物连接配置") -> ("启用"=w208:bool, "连接类型"=w207:enum16{"串口", "TCP"}, "串口"=w206:string, "IP"=w205:string, "PORT"=w204:string)
                    n218 = global write "系统设置全局变量.vi" "CODcr模块版本"("CODcr模块版本") -> ()
                    n219 = global write "系统设置全局变量.vi" "进样类型"("进样类型") -> ()
                    n220 = global write "系统设置全局变量.vi" "加标回收模块版本"("加标回收模块版本") -> ()
                    n221 = global write "系统设置全局变量.vi" "SYSTEM Interface.总磷总氮类型"("模块配置类型") -> ()
                    n222 = Unbundle By Name("CODcr连接配置") -> ("启用"=w267:bool, "连接类型"=w227:enum16{"串口", "TCP"}, "串口"=w226:string, "IP"=w225:string, "PORT"=w224:string, "波特率"=w196:u32)
                    n223 = global write "系统设置全局变量.vi" "氨氮模块版本"("氨氮模块版本") -> ()
                    n224 = global write "系统设置全局变量.vi" "启用运维打卡"("运维打卡启用") -> ()
                    n225 = case shown="\"通用流路版本\"" w247 {
                      tunnel: "CODMn连接配置" -> [w324 w330 w336]
                      frame "PLC版", Default {
                        n226 = global read "CODMn断电保存全局变量.vi" "Serial Config"() -> (w319:T21)
                        n227 = Unbundle By Name(w324) -> ("连接类型"=w323:enum16{"串口", "TCP"}, "串口"=w322:string, "IP"=w321:string, "PORT"=w320:string, "波特率"=w317:u32)
                        n228 = Bundle By Name(cluster=w319, "baud rate (bps)"=w317) -> (w318:T21)
                        n229 = global write "CODMn断电保存全局变量.vi" "MB通信方式选择"(w323) -> ()
                        n230 = global write "CODMn断电保存全局变量.vi" "VISA resource name"(w322) -> ()
                        n231 = global write "CODMn断电保存全局变量.vi" "IP"(w321) -> ()
                        n232 = global write "CODMn断电保存全局变量.vi" "PORT"(w320) -> ()
                        n233 = global write "CODMn断电保存全局变量.vi" "Serial Config"(w318) -> ()
                      }
                      frame "单片机版" {
                        n234 = Unbundle By Name(w330) -> ("连接类型"=w326:enum16{"串口", "TCP"}, "串口"=w327:string, "IP"=w328:string, "PORT"=w329:string, "波特率"=w325:u32)
                        n235 = global write "CODMn断电保存全局变量.vi" "波特率"(w325) -> ()
                        n236 = global write "CODMn断电保存全局变量.vi" "MB通信方式选择"(w326) -> ()
                        n237 = global write "CODMn断电保存全局变量.vi" "VISA Resource"(w327) -> ()
                        n238 = global write "CODMn断电保存全局变量.vi" "IP"(w328) -> ()
                        n239 = global write "CODMn断电保存全局变量.vi" "PORT"(w329) -> ()
                      }
                      frame "通用流路版本" {
                        n240 = Unbundle By Name(w336) -> ("连接类型"=w335:enum16{"串口", "TCP"}, "串口"=w334:string, "波特率"=w333:u32, "IP"=w332:string, "PORT"=w331:string)
                        n241 = global write "总磷总氮断电保存全局变量.vi" "MB通信方式选择"(w335) -> ()
                        n242 = global write "总磷总氮断电保存全局变量.vi" "VISA Resource"(w334) -> ()
                        n243 = global write "总磷总氮断电保存全局变量.vi" "波特率"(w333) -> ()
                        n244 = global write "总磷总氮断电保存全局变量.vi" "PORT"(w331) -> ()
                        n245 = global write "总磷总氮断电保存全局变量.vi" "IP"(w332) -> ()
                      }
                    }
                    n246 = Unbundle By Name("CODMn连接配置") -> ("启用"=w266:bool)
                    n247 = global write "系统设置全局变量.vi" "河水净化启用"("河水净化启用") -> ()
                    n248 = global write "系统设置全局变量.vi" "多参数模块版本"("多参数模块版本") -> ()
                    n249 = global write "系统设置全局变量.vi" "流量计启用"("流量计启用") -> ()
                    n250 = global write "系统设置全局变量.vi" "总氮模块版本"("总氮模块版本") -> ()
                    n251 = global write "系统设置全局变量.vi" "CODMn模块版本"("CODMn模块版本") -> ()
                    n252 = global write "系统设置全局变量.vi" "采配水模块类型"("采配水模块类型") -> ()
                    n253 = Unbundle By Name("总磷连接配置") -> ("启用"=w264:bool, "连接类型"=w241:enum16{"串口", "TCP"}, "串口"=w240:string, "IP"=w239:string, "PORT"=w238:string, "波特率"=w195:u32)
                    n254 = global write "系统设置全局变量.vi" "设备类型"("设备类型") -> ()
                    n255 = global write "系统设置全局变量.vi" "总磷模块版本"("总磷模块版本") -> ()
                    n256 = Unbundle By Name("氨氮连接配置") -> ("启用"=w263:bool, "连接类型"=w245:enum16{"串口", "TCP"}, "串口"=w244:string, "IP"=w243:string, "PORT"=w242:string, "波特率"=w194:u32)
                    n257 = Unbundle By Name("总氮连接配置") -> ("启用"=w265:bool, "连接类型"=w237:enum16{"串口", "TCP"}, "串口"=w236:string, "IP"=w235:string, "PORT"=w234:string, "波特率"=w193:u32)
                    n258 = Unbundle By Name("加标回收连接配置") -> ("启用"=w269:bool, "连接类型"=w232:enum16{"串口", "TCP"}, "串口"=w233:string, "IP"=w230:string, "PORT"=w229:string)
                    n259 = Unbundle By Name("多参数连接配置") -> ("启用"=w268:bool, "连接类型"=w223:enum16{"串口", "TCP"}, "串口"=w222:string, "IP"=w221:string, "PORT"=w220:string)
                    n260 = global write "非断电保持全局变量.vi" "数据库类型"("数据库类型") -> ()
                    n261 = global write "系统设置全局变量.vi" "氟化物启用"(w208) -> ()
                    n262 = global write "总磷总氮断电保存全局变量.vi" "MB通信方式选择"(w207) -> ()
                    n263 = global write "总磷总氮断电保存全局变量.vi" "VISA Resource"(w206) -> ()
                    n264 = global write "总磷总氮断电保存全局变量.vi" "IP"(w205) -> ()
                    n265 = global write "总磷总氮断电保存全局变量.vi" "PORT"(w204) -> ()
                    n266 = global write "系统设置全局变量.vi" "CODcr启用"(w267) -> ()
                    n267 = global write "总磷总氮断电保存全局变量.vi" "MB通信方式选择"(w227) -> ()
                    n268 = global write "总磷总氮断电保存全局变量.vi" "VISA Resource"(w226) -> ()
                    n269 = global write "总磷总氮断电保存全局变量.vi" "IP"(w225) -> ()
                    n270 = global write "总磷总氮断电保存全局变量.vi" "PORT"(w224) -> ()
                    n271 = global write "系统设置全局变量.vi" "CODMn启用"(w266) -> ()
                    n272 = local read "总磷模块版本"() -> (w214:T4)
                    n273 = global write "系统设置全局变量.vi" "总磷总氮启用"(w264) -> ()
                    n274 = local read "氨氮模块版本"() -> (w213:T4)
                    n275 = global write "系统设置全局变量.vi" "氨氮启用"(w263) -> ()
                    n276 = local read "总氮模块版本"() -> (w212:T4)
                    n277 = global write "系统设置全局变量.vi" "总氮启用"(w265) -> ()
                    n278 = global write "系统设置全局变量.vi" "质控单元启用"(w269) -> ()
                    n279 = global write "系统设置全局变量.vi" "多参数启用"(w268) -> ()
                    n280 = global write "总磷总氮断电保存全局变量.vi" "波特率"(w196) -> ()
                    n281 = To Unsigned Word Integer(number=w232) -> (unsigned 16bit integer=w231:u16)
                    n282 = case shown="\"V3\"" w214 {
                      tunnel: w241 -> [w311 w316]
                      tunnel: w240 -> [w310 w315]
                      tunnel: w239 -> [w309 w314]
                      tunnel: w238 -> [w308 w313]
                      tunnel: w195 -> [w307 w312]
                      frame "V2", Default {
                        n283 = global write "总磷总氮断电保存全局变量.vi" "MB通信方式选择"(w311) -> ()
                        n284 = global write "总磷总氮断电保存全局变量.vi" "VISA Resource"(w310) -> ()
                        n285 = global write "总磷总氮断电保存全局变量.vi" "IP"(w309) -> ()
                        n286 = global write "总磷总氮断电保存全局变量.vi" "PORT"(w308) -> ()
                        n287 = global write "总磷总氮断电保存全局变量.vi" "波特率"(w307) -> ()
                      }
                      frame "V3" {
                        n288 = global write "总磷总氮断电保存全局变量.vi" "MB通信方式选择"(w316) -> ()
                        n289 = global write "总磷总氮断电保存全局变量.vi" "VISA Resource"(w315) -> ()
                        n290 = global write "总磷总氮断电保存全局变量.vi" "IP"(w314) -> ()
                        n291 = global write "总磷总氮断电保存全局变量.vi" "PORT"(w313) -> ()
                        n292 = global write "总磷总氮断电保存全局变量.vi" "波特率"(w312) -> ()
                      }
                    }
                    n293 = case shown="\"V2\", Default" w213 {
                      tunnel: w245 -> [w298 w306]
                      tunnel: w244 -> [w299 w305]
                      tunnel: w243 -> [w300 w304]
                      tunnel: w242 -> [w301 w303]
                      tunnel: w194 -> [w297 w302]
                      frame "V2", Default {
                        n294 = global write "总磷总氮断电保存全局变量.vi" "MB通信方式选择"(w298) -> ()
                        n295 = global write "总磷总氮断电保存全局变量.vi" "VISA Resource"(w299) -> ()
                        n296 = global write "总磷总氮断电保存全局变量.vi" "IP"(w300) -> ()
                        n297 = global write "总磷总氮断电保存全局变量.vi" "PORT"(w301) -> ()
                        n298 = global write "总磷总氮断电保存全局变量.vi" "波特率"(w297) -> ()
                      }
                      frame "V3" {
                        n299 = global write "总磷总氮断电保存全局变量.vi" "MB通信方式选择"(w306) -> ()
                        n300 = global write "总磷总氮断电保存全局变量.vi" "VISA Resource"(w305) -> ()
                        n301 = global write "总磷总氮断电保存全局变量.vi" "IP"(w304) -> ()
                        n302 = global write "总磷总氮断电保存全局变量.vi" "PORT"(w303) -> ()
                        n303 = global write "总磷总氮断电保存全局变量.vi" "波特率"(w302) -> ()
                      }
                    }
                    n304 = case shown="\"V3\"" w212 {
                      tunnel: w237 -> [w291 w296]
                      tunnel: w236 -> [w290 w295]
                      tunnel: w235 -> [w289 w294]
                      tunnel: w234 -> [w288 w293]
                      tunnel: w193 -> [w287 w292]
                      frame "V2", Default {
                        n305 = global write "总磷总氮断电保存全局变量.vi" "MB通信方式选择"(w291) -> ()
                        n306 = global write "总磷总氮断电保存全局变量.vi" "VISA Resource"(w290) -> ()
                        n307 = global write "总磷总氮断电保存全局变量.vi" "IP"(w289) -> ()
                        n308 = global write "总磷总氮断电保存全局变量.vi" "PORT"(w288) -> ()
                        n309 = global write "总磷总氮断电保存全局变量.vi" "波特率"(w287) -> ()
                      }
                      frame "V3" {
                        n310 = global write "总磷总氮断电保存全局变量.vi" "MB通信方式选择"(w296) -> ()
                        n311 = global write "总磷总氮断电保存全局变量.vi" "VISA Resource"(w295) -> ()
                        n312 = global write "总磷总氮断电保存全局变量.vi" "IP"(w294) -> ()
                        n313 = global write "总磷总氮断电保存全局变量.vi" "PORT"(w293) -> ()
                        n314 = global write "总磷总氮断电保存全局变量.vi" "波特率"(w292) -> ()
                      }
                    }
                    n315 = Decimal String To Number(string=w229) -> (number=w228:i32)  [unwired: 2 in, 1 out]
                    n316 = Decimal String To Number(string=w220) -> (number=w219:i32)  [unwired: 2 in, 1 out]
                    n317 = local read "加标回收模块版本"() -> (w211:T2)
                    n318 = local read "多参数模块版本"() -> (w210:T3)
                    n319 = case shown="\"V2\"" w211 {
                      tunnel: w233 -> [w276 w280 w286]
                      tunnel: w231 -> [w278 w282 w285]
                      tunnel: w230 -> [w275 w279 w284]
                      tunnel: w228 -> [w277 w281 w283]
                      frame "V1", Default {
                        n320 = global write "ZK断电保存全局变量.vi" "Type"(w278) -> ()
                        n321 = global write "ZK断电保存全局变量.vi" "COM Port"(w276) -> ()
                        n322 = global write "ZK断电保存全局变量.vi" "IP Address"(w275) -> ()
                        n323 = global write "ZK断电保存全局变量.vi" "TCP_Port"(w277) -> ()
                      }
                      frame "V2" {
                        n324 = global write "ZK断电保存全局变量.vi" "Type"(w282) -> ()
                        n325 = global write "ZK断电保存全局变量.vi" "COM Port"(w280) -> ()
                        n326 = global write "ZK断电保存全局变量.vi" "IP Address"(w279) -> ()
                        n327 = global write "ZK断电保存全局变量.vi" "TCP_Port"(w281) -> ()
                      }
                      frame "V4" {
                        n328 = global write "ZK断电保存全局变量.vi" "Type"(w285) -> ()
                        n329 = global write "ZK断电保存全局变量.vi" "COM Port"(w286) -> ()
                        n330 = global write "ZK断电保存全局变量.vi" "IP Address"(w284) -> ()
                        n331 = global write "ZK断电保存全局变量.vi" "TCP_Port"(w283) -> ()
                      }
                    }
                    n332 = case shown="\"集成式多参\"" w210 {
                      tunnel: w223 -> [_ w274]
                      tunnel: w222 -> [w270 w273]
                      tunnel: w221 -> [_ w272]
                      tunnel: w219 -> [_ w271]
                      frame "原位多参数", Default {
                        n333 = global write "多参数断电保存全局变量.vi" "VISA Resource"(w270) -> ()
                      }
                      frame "集成式多参" {
                        n334 = global write "断电保存变量.vi" "连接方式"(w274) -> ()
                        n335 = global write "断电保存变量.vi" "VISA资源名称"(w273) -> ()
                        n336 = global write "断电保存变量.vi" "IP"(w272) -> ()
                        n337 = global write "断电保存变量.vi" "Port"(w271) -> ()
                      }
                    }
                  }
                  frame #1 {
                    n338 = call <vilib>:"Application Directory.vi"() -> ("Application Directory"=w353:path)
                    n339 = Build Path(base path=w353, name or relative path="data\\sys.ini" ("名称或相对路径")) -> (appended path=w351:path)
                    n340 = call <vilib>:"Open Config Data.vi"("configuration file path"=w351) -> ("error out"=w349:errorcluster, "refnum"=w350:T26)  [unwired: 8 in, 1 out]
                    n341 = vi-ref "系统设置全局变量.vi"() -> (w362:refnum<vi>)
                    n342 = call <userlib>:"Write Panel to INI__ogtk.vi"("error in (no error)"=w349, "VI ref"=w362, "refnum"=w350) -> ("error out"=w360:errorcluster, "refnum out"=w361:T26)  [unwired: 7 in]
                    n343 = call <vilib>:"Close Config Data.vi"("error in (no error)"=w360, "refnum"=w361) -> ("error out"=w355:errorcluster, "file path"=w354:path)  [unwired: 8 in]
                    n344 = Open/Create/Replace File(file path (use dialog)=w354, error in=w355) -> (refnum out=w358:refnum<file>, error out=w359:errorcluster)  [unwired: 4 in, 1 out]
                    n345 = Flush File(refnum=w358, error in=w359) -> (refnum out=w357:refnum<file>, error out=w356:errorcluster)
                    n346 = Close File(refnum=w357, error in=w356) -> (error out=w344:errorcluster)  [unwired: 1 out]
                    n347 = global read "系统设置全局变量.vi" "氨氮模块版本"() -> (w343:T4)
                    n348 = case shown="\"V3\"" w343 {
                      tunnel: [w381 w384] -> w348
                      tunnel: w344 -> [w382 w383]
                      frame "V2", Default {
                        n349 = call "配置写入.vi"("error in (no error)"=w382) -> ("错误输出"=w381:errorcluster)  [unwired: 10 in]
                      }
                      frame "V3" {
                        n350 = call "仪器配置写入.vi"("error in (no error)"=w383) -> ("错误输出"=w384:errorcluster)  [unwired: 10 in]
                      }
                    }
                    n351 = global read "系统设置全局变量.vi" "总磷模块版本"() -> (w342:T4)
                    n352 = case shown="\"V2\", Default" w342 {
                      tunnel: w348 -> [w378 w380]
                      tunnel: [w377 w379] -> w347
                      frame "V2", Default {
                        n353 = call "配置写入.vi"("error in (no error)"=w378) -> ("错误输出"=w377:errorcluster)  [unwired: 10 in]
                      }
                      frame "V3" {
                        n354 = call "仪器配置写入.vi"("error in (no error)"=w380) -> ("错误输出"=w379:errorcluster)  [unwired: 10 in]
                      }
                    }
                    n355 = global read "系统设置全局变量.vi" "总氮模块版本"() -> (w341:T4)
                    n356 = case shown="\"V2\", Default" w341 {
                      tunnel: w347 -> [w373 w376]
                      tunnel: [w374 w375] -> w346
                      frame "V2", Default {
                        n357 = call "配置写入.vi"("error in (no error)"=w373) -> ("错误输出"=w374:errorcluster)  [unwired: 10 in]
                      }
                      frame "V3" {
                        n358 = call "仪器配置写入.vi"("error in (no error)"=w376) -> ("错误输出"=w375:errorcluster)  [unwired: 10 in]
                      }
                    }
                    n359 = call "仪器配置写入.vi"("error in (no error)"=w346) -> ("错误输出"=w345:errorcluster)  [unwired: 10 in]
                    n360 = global read "系统设置全局变量.vi" "加标回收模块版本"() -> (w340:T2)
                    n361 = case shown="\"V2\"" w340 {
                      tunnel: w345 -> [w368 w370 w372]
                      tunnel: [w367 w369 w371] -> w339
                      frame "V1", Default {
                        n362 = call "配置信息写入.vi"("error in (no error)"=w368) -> ("error out"=w367:errorcluster)  [unwired: 10 in]
                      }
                      frame "V4" {
                        n363 = call "配置信息写入.vi"("error in (no error)"=w370) -> ("error out"=w369:errorcluster)  [unwired: 10 in]
                      }
                      frame "V2" {
                        n364 = call "配置信息写入.vi"("error in (no error)"=w372) -> ("error out"=w371:errorcluster)  [unwired: 10 in]
                      }
                    }
                    n365 = global read "系统设置全局变量.vi" "多参数模块版本"() -> (w338:T3)
                    n366 = case shown="\"集成式多参\"" w338 {
                      tunnel: w339 -> [w365 w366]
                      tunnel: [w364 w366] -> w337
                      frame "原位多参数", Default {
                        n367 = call "配置保存.vi"("error in (no error)"=w365) -> ("error out"=w364:errorcluster)  [unwired: 10 in]
                      }
                      frame "集成式多参" {
                        n368 = call "配置文件保存.vi"() -> ()  [unwired: 12 in]
                      }
                    }
                    n369 = case shown="No Error" w337 {
                      frame No Error {
                        n370 = global read "系统设置全局变量.vi" "CODMn模块版本"() -> (w363:T9)
                        n371 = case shown="\"通用流路版本\"" w363 {
                          frame "PLC版", Default {
                            n372 = call "配置文件保存.vi"() -> ()  [unwired: 12 in]
                          }
                          frame "单片机版" {
                            n373 = call "配置文件保存.vi"() -> ()  [unwired: 12 in]
                          }
                          frame "通用流路版本" {
                            n374 = call "仪器配置写入.vi"() -> ()  [unwired: 11 in, 1 out]
                          }
                        }
                      }
                      frame Error {
                      }
                    }
                  }
                  frame #2 {
                    n375 = disable-structure shown="RUN_TIME_ENGINE==True" {
                      frame condition #0 (active) {
                      }
                      frame condition #1 {
                        (unwired) "cmd /c taskkill /f /im %s & ping 127.0.0.1 -n 5 & \"%s\"" ("格式字符串")
                        n376 = control-ref of="该应用程序"() -> (w391:refnum<vi>)
                        n377 = property class="App"(reference=w391) -> ("App.Name"=w387:string)  [unwired: 1 in, 2 out]
                        n378 = Format Into String(format string="cmd /c taskkill /f /im %s" ("格式字符串"), w387) -> (resulting string=w389:string)  [unwired: 2 in, 1 out]
                        n379 = call <vilib>:"Application Directory.vi"() -> ("Application Directory"=w388:path)
                        n380 = call <vilib>:"System Exec.vi"("run minimized? (F)"=TRUE, "wait until completion? (T)"=FALSE, "working directory"=w388, "command line"=w389) -> ()  [unwired: 4 in, 4 out]
                      }
                    }
                  }
                }
              }
            }
          }
          event Value Change {
            n381 = event-data() -> ("NewVal"=w392:T11)  [unwired: 1 in, 5 out]
            n382 = case shown="\"氨氮总磷二合一模块\"" w392 {
              frame "单模块", Default {
              }
              frame "总磷总氮二合一模块" {
                n383 = property on="启用" class="Bool (strict)"("Value"=FALSE ("值")) -> ()  [unwired: 2 in, 2 out]
              }
              frame "氨氮总磷二合一模块" {
                n384 = property on="启用" class="Bool (strict)"("Value"=FALSE ("值")) -> ()  [unwired: 2 in, 2 out]
                n385 = property on="启用" class="Bool (strict)"("Value"=FALSE ("值")) -> ()  [unwired: 2 in, 2 out]
              }
            }
          }
          event Value Change {
            n386 = event-data() -> ("NewVal"=w396:bool)  [unwired: 1 in, 5 out]
            n387 = case shown="False" w396 {
              frame False {
                n388 = property on="加标回收模块版本" class="Enum (strict)"("Value"=加标回收模块版本."V4" ("加标回收模块版本")) -> ()  [unwired: 2 in, 2 out]
              }
              frame True {
                n389 = property on="加标回收模块版本" class="Enum (strict)"() -> ("Value"=w398:T2)  [unwired: 2 in, 2 out]
                n390 = case shown="\"V2\"" w398 {
                  frame "V1", Default {
                    n391 = property on="进样类型" class="Clust (strict)"("Value"=T12 {"氨氮采样杯采样"=FALSE, "总磷采样杯采样"=FALSE, "总氮采样杯采样"=FALSE, "CODMn采样杯采样"=FALSE, "CODcr采样杯采样"=FALSE, "氟化物采样杯采样"=FALSE, "氟化物采样杯采样 2"=FALSE} ("进样类型")) -> ()  [unwired: 2 in, 2 out]
                  }
                  frame "V2" {
                    n392 = property on="进样类型" class="Clust (strict)"("Value"=T12 {"氨氮采样杯采样"=TRUE, "总磷采样杯采样"=TRUE, "总氮采样杯采样"=TRUE, "CODMn采样杯采样"=TRUE, "CODcr采样杯采样"=TRUE, "氟化物采样杯采样"=TRUE, "氟化物采样杯采样 2"=FALSE} ("进样类型")) -> ()  [unwired: 2 in, 2 out]
                  }
                  frame "V4" {
                  }
                }
              }
            }
          }
          event Value Change {
            n393 = event-data() -> ("NewVal"=w401:T2)  [unwired: 1 in, 5 out]
            n394 = case shown="\"V1\", Default" w401 {
              frame "V1", Default {
                n395 = property on="进样类型" class="Clust (strict)"("Value"=T12 {"氨氮采样杯采样"=FALSE, "总磷采样杯采样"=FALSE, "总氮采样杯采样"=FALSE, "CODMn采样杯采样"=FALSE, "CODcr采样杯采样"=FALSE, "氟化物采样杯采样"=FALSE, "氟化物采样杯采样 2"=FALSE} ("进样类型")) -> ()  [unwired: 2 in, 2 out]
              }
              frame "V2" {
                n396 = property on="进样类型" class="Clust (strict)"("Value"=T12 {"氨氮采样杯采样"=TRUE, "总磷采样杯采样"=TRUE, "总氮采样杯采样"=TRUE, "CODMn采样杯采样"=TRUE, "CODcr采样杯采样"=TRUE, "氟化物采样杯采样"=TRUE, "氟化物采样杯采样 2"=FALSE} ("进样类型")) -> ()  [unwired: 2 in, 2 out]
              }
              frame "V4" {
              }
            }
          }
        }
      }
    }
  }
